vi "Sort 2D String Arrays.vi"(4 "Arrays in":string[][](array[string])) -> (1 "Arrays out":string[][](array[string]))   [LabVIEW 2013]
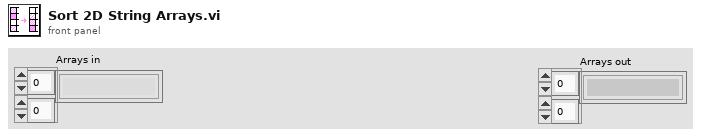
[diagram p1: front panel]
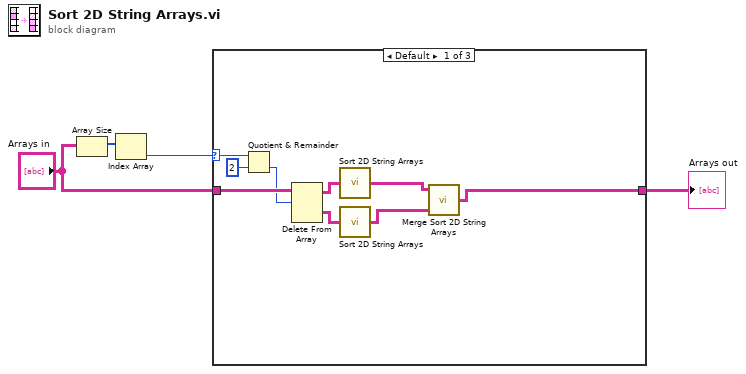
[diagram p0: block diagram]
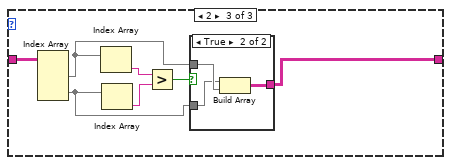
[diagram p3: hidden frame]
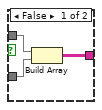
[diagram p4: hidden frame]
diagram:
  n1 = Array Size(array="Arrays in") -> (size(s)=w4:i32[])
  n2 = Index Array(array=w4) -> (element=w1:i32)  [unwired: 1 in]
  n3 = case shown="Default" w1 {
    selector: w1 -> [w12 _ _]
    tunnel: "Arrays in" -> [w13 w14 w21]
    tunnel: [w5 w14 w15] -> w2
    frame Default {
      n4 = Quotient & Remainder(x=w12, y=2) -> (floor(x/y)=w10:i32)  [unwired: 1 out]
      n5 = Delete From Array(array=w13, length=w10) -> (deleted portion=w8:string[][], array with subset deleted=w9:string[][])  [unwired: 2 in]
      n6 = call "Sort 2D String Arrays.vi"("Arrays in"=w9) -> ("Arrays out"=w7:string[][])  [unwired: 4 in]
      n7 = call "Sort 2D String Arrays.vi"("Arrays in"=w8) -> ("Arrays out"=w6:string[][])  [unwired: 4 in]
      n8 = call "Merge Sort 2D String Arrays.vi"("2D String Array A"=w7, "2D String Array B"=w6) -> ("Sorted 2D String Array"=w5:string[][])  [unwired: 5 in]
    }
    frame 1 {
    }
    frame 2 {
      n9 = Index Array(array=w21) -> (element #1=w17:string[], element #2=w16:string[])  [unwired: 4 in]
      n10 = Index Array(array=w17) -> (element=w19:string)  [unwired: 1 in]
      n11 = Index Array(array=w16) -> (element=w18:string)  [unwired: 1 in]
      n12 = Greater?(x=w19, y=w18) -> (0:w20:bool)
      n13 = case shown="True" w20 {
        tunnel: w17 -> [w24 w27]
        tunnel: w16 -> [w23 w26]
        tunnel: [w22 w25] -> w15
        frame False {
          n14 = Build Array(w24, w23) -> (w22:string[][])
        }
        frame True {
          n15 = Build Array(w26, w27) -> (w25:string[][])
        }
      }
    }
  }
  "Arrays out" <- w2
